vi "29931_load_curve.vi"() -> ()   [LabVIEW 2017]
uses:
  <vilib>/Utility/file.llb/Read Delimited Spreadsheet (DBL).vi
  <instrlib>/Lake Shore Cryotronics 370/Lake Shore Cryotronics 370.lvlib
panel:
  out "n_points":i32
  out "size(s)":i32[](array[numeric])
  out "R":dbl
  out "temp":dbl
  out "all rows":dbl[][](array[numeric]) format="%0.3f"
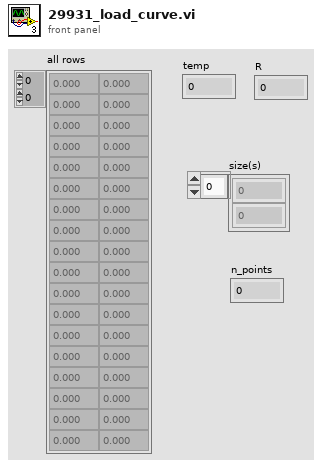
[diagram p1: front panel]
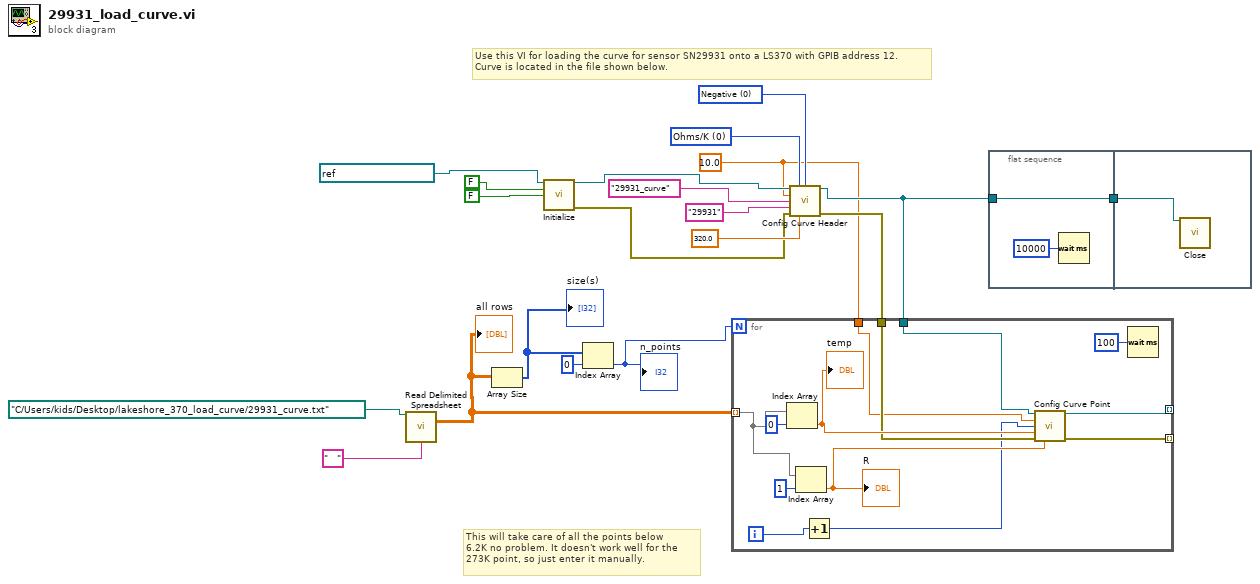
[diagram p0: block diagram]
diagram:
  w12 = u16 0 items=["Negative", "Positive"] ("Temp Coefficient (0: Negative)")
  w14 = u16 0 items=["Ohms/K", "Log Ohms/K"] ("Curve Data Format (0: Ohms/K)")
  w5 = 10.0 ("Curve (1)")
  # "Use this VI for loading the curve for sensor SN29931 onto a LS370 with GPIB address 12.\nCurve is located in the file shown below."
  # "This will take care of all the points below\n6.2K no problem. It doesn't work well for the\n273K point, so just enter it manually."
  n1 = call-poly <vilib>:"Read Delimited Spreadsheet.vi"("file path (dialog if empty)"=path "C:/Users/kids/Desktop/lakeshore_370_load_curve/29931_curve.txt", "delimiter (\\t)"="   " ("delimiter (\\t)")) -> ("all rows"=w4:dbl[][])  [unwired: 8 in, 5 out]
  "all rows" <- w4
  n2 = Array Size(array=w4) -> (size(s)=w3:i32[])
  "size(s)" <- w3
  n3 = call <instrlib>:"Initialize.vi"("VISA resource name"=refnum<visa-resource-name> "GPIB0::12::INSTR", "ID Query (True)"=FALSE, "Reset (True)"=FALSE) -> ("VISA resource name out"=w11:refnum<visa-resource-name>, "error out"=w10:errorcluster)  [unwired: 11 in]
  n4 = Index Array(array=w3, index=0) -> (element=w1:i32)
  "n_points" <- w1
  n5 = call <instrlib>:"Config Curve Header.vi"("VISA resource name"=w11, "Curve Data Format (0: Ohms/K)"=w14, "Temp Coefficient (0: Negative)"=w12, "Curve (1)"=w5, "Curve Name (\"\")"="29931_curve" ("Curve Name (\"\")"), "Curve Serial Number (\"\")"="29931" ("Curve Serial Number (\"\")"), "error in (no error)"=w10, "Limit Value (0.000)"=320.0) -> ("VISA resource name out"=w9:refnum<visa-resource-name>, "error out"=w8:errorcluster)  [unwired: 6 in]
  n6 = for {
    N: w1 -> [_]
    tunnel: w4 -> [w31] mode=indexing
    tunnel: w9 -> [w28]
    tunnel: w8 -> [w26]
    tunnel: w5 -> [w24]
    tunnel: [w22] -> _ mode=indexing
    tunnel: [w21] -> _ mode=indexing
    i -> [w29]
    n7 = Index Array(array=w31, index=0) -> (element=w27:dbl)
    "temp" <- w27
    n8 = Index Array(array=w31, index=1) -> (element=w25:dbl)
    "R" <- w25
    n9 = Increment(x=w29) -> (x+1=w23:i32)
    n10 = call <instrlib>:"Config Curve Point.vi"("VISA resource name"=w28, "Curve (1)"=w24, "Index (1)"=w23, "Temperature Value (0.0000)"=w27, "error in (no error)"=w26, "Units Value (0.00000)"=w25) -> ("VISA resource name out"=w22:refnum<visa-resource-name>, "error out"=w21:errorcluster)  [unwired: 8 in]
    n11 = Wait (ms)(milliseconds to wait=u32 100) -> ()  [unwired: 1 out]
  }
  n12 = flat-sequence {
    tunnel: w9 -> [w35]
    tunnel: [w35] -> w20
    tunnel: w20 -> [w36]
    frame #0 {
      n13 = Wait (ms)(milliseconds to wait=u32 10000) -> ()  [unwired: 1 out]
    }
    frame #1 {
      n14 = call <instrlib>:"Close.vi"("VISA resource name"=w36) -> ()  [unwired: 14 in, 1 out]
    }
  }
